vi "Add Standard Regex Router.vi"(10 "Controller Map":T1, 11 "Route Handler Map In":T3) -> (3 "Route Handler Map":T3)   [LabVIEW 2020, in "HTTP Server.lvlib" / "Server.lvclass"]
uses:
  Server.lvclass
  Route Handler Map.ctl
  Priority.ctl
  Route Handler/Route Handler.lvclass
  Controller Map.ctl
  Controller/Controller.lvclass
  PathRegex Router/PathRegex Router.lvclass
  C:/dev/IlluminatedG/lv-http-server/HTTP Server/Route Handler/Route Handler.lvclass
  Server.lvclass/Server.ctl
  HTTP Server.lvlib
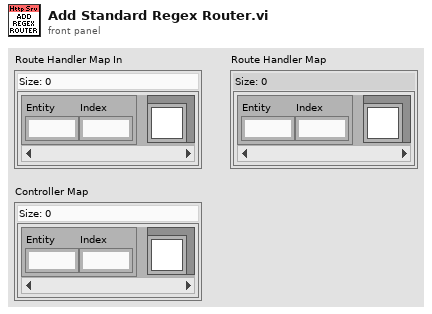
[diagram p1: front panel]
types:
  T1 = typedef "HTTP Server.lvlib/Controller Map.ctl" = map{T2, refnum<class "Controller.lvclass">}
  T2 = typedef "HTTP Server.lvlib/Priority.ctl" = cluster{"Entity":u16, "Index":u16}
  T3 = typedef "HTTP Server.lvlib/Route Handler Map.ctl" = map{T2, refnum<class "Route Handler.lvclass">}
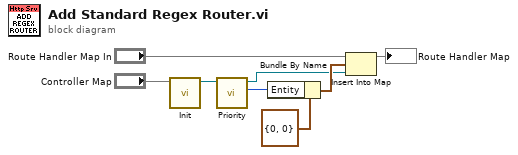
[diagram p0: block diagram]
diagram:
  n1 = call "Init.vi"("Controller Map"="Controller Map") -> ("PathRegex Router out"=w7:refnum<class "PathRegex Router.lvclass">)  [unwired: 9 in, 1 out]
  n2 = call-dynamic "Priority.vi"("PathRegex Router in"=w7) -> ("Priority"=w5:u16, "PathRegex Router out"=w2:refnum<class "PathRegex Router.lvclass">)  [unwired: 8 in, 1 out]
  n3 = Bundle By Name(cluster=T2 {"Entity"=0, "Index"=0} ("Priority"), "Entity"=w5) -> (w3:T2)
  n4 = Insert Into Map(map in="Route Handler Map In", key=w3, value=w2) -> (map out=→"Route Handler Map":T3)  [unwired: 2 out]
